vi "detectISOSPI.vi"(8 "errin":errorcluster, 11 "VISA resource name":refnum<visa-resource-name>) -> (0 "sortie d'erreur":errorcluster caption="errout", 3 "cas faux":string)   [LabVIEW 2020]
uses:
  <vilib>/Instr/_visa.llb/VISA Configure Serial Port (Instr).vi
panel:
  out "buffer de lecture":string
  # "2A49 444E 3F0A"
  # "*IDN?"
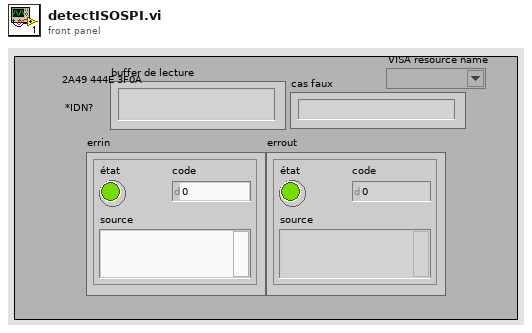
[diagram p1: front panel]
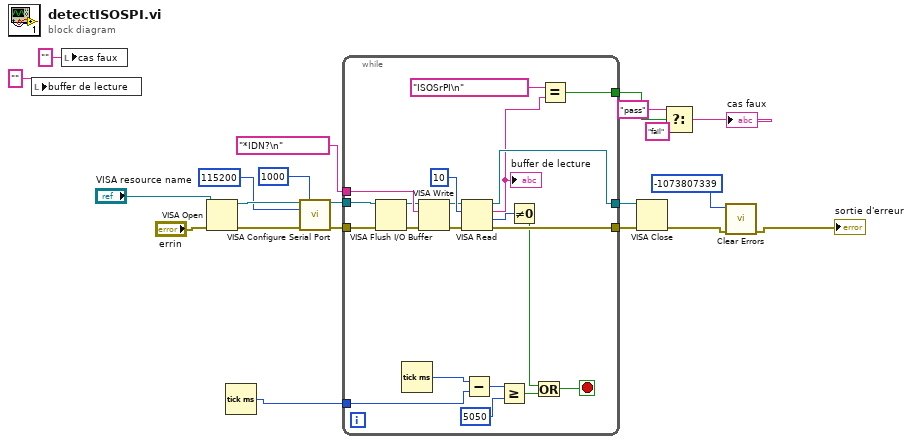
[diagram p0: block diagram]
diagram:
  n1 = local write "buffer de lecture"("" ("buffer de lecture")) -> ()
  n2 = local write "cas faux"("" ("cas faux")) -> ()
  n3 = VISA Open(error in (no error)="errin", VISA resource name="VISA resource name") -> (VISA resource name=w14:refnum<visa-resource-name>, error out=w13:errorcluster)  [unwired: 3 in]
  n4 = Tick Count (ms)() -> (millisecond timer value=w3:u32)
  n5 = call-poly "VISA Configure Serial Port"("VISA resource name"=w14, "timeout (10sec)"=u32 1000, "baud rate (9600)"=u32 115200, "error in (no error)"=w13) -> ("VISA resource name out"=w9:refnum<visa-resource-name>, "error out"=w11:errorcluster)  [unwired: 10 in]
  n6 = while {
    tunnel: [w42] -> w15
    tunnel: w11 -> [w34]
    tunnel: "*IDN?\n" ("buffer d'écriture") -> [w39]
    tunnel: w9 -> [w35]
    tunnel: [w37] -> w8
    tunnel: [w29] -> w6
    tunnel: w3 -> [w27]
    stop <- w22 stop-if-true
    n7 = VISA Flush I/O Buffer(VISA resource name=w35, error in (no error)=w34) -> (VISA resource name out=w32:refnum<visa-resource-name>, error out=w33:errorcluster)  [unwired: 1 in]
    n8 = Tick Count (ms)() -> (millisecond timer value=w28:u32)
    n9 = VISA Write(VISA resource name=w32, write buffer=w39, error in (no error)=w33) -> (VISA resource name out=w36:refnum<visa-resource-name>, error out=w38:errorcluster)  [unwired: 1 out]
    n10 = VISA Read(VISA resource name=w36, byte count=u32 10 ("nombre d'octets"), error in (no error)=w38) -> (VISA resource name out=w37:refnum<visa-resource-name>, read buffer=w31:string, return count=w40:u32, error out=w42:errorcluster)
    "buffer de lecture" <- w31
    n11 = Subtract(x=w28, y=w27) -> (x-y=w26:u32)
    n12 = Greater Or Equal? ("Supérieur ou égal ?")(x=w26, y=u32 5050) -> (x >= y?=w24:bool)
    n13 = Not Equal To 0?(x=w40) -> (x != 0?=w23:bool)
    n14 = Or(x=w23, y=w24) -> (x .or. y?=w22:bool)
    n15 = Equal? ("Égaux ?")(x="ISOSrPI\n", y=w31) -> (x = y?=w29:bool)
  }
  n16 = VISA Close(VISA resource name=w8, error in (no error)=w15) -> (error out=w5:errorcluster)
  n17 = Select ("Sélectionner")(t="pass", s=w6, f="fail" ("cas faux")) -> (s? t:f=→"cas faux":string)
  n18 = call <vilib>:"Clear Errors.vi"("error in (no error)"=w5, "specific error code to clear (0: all)"=-1073807339) -> ("error out"=→"sortie d'erreur":errorcluster)  [unwired: 4 in, 1 out]
